vi "High Resolution Wait.vi"(8 "error in (no error)":errorcluster, 11 "wait time (s)":dbl format="%#_6p") -> (0 "error out":errorcluster)   [LabVIEW 2020]
doc: "LabVIEW no longer supports this VI. Use the High Resolution Polling Wait VI instead.\n\nWaits the specified time. Use this VI when you need higher resolution of wait time than you can obtain with the Wait (ms) function. \n\nThe time resolution of this VI may vary with different operating systems and CPU types.\n\nUnlike the Wait (ms) function, this VI does not yield. If <b>wait time</b> is less than 1 to 2 ms, this VI polls in a tight loop. If <b>wait time</b> is greater than 1 to 2 ms, this VI polls in a tight loop for the last 1 to 2 ms."
panel:
  # "This VI is deprecated. Use the following VI instead:\n\nvi.lib\\Utility\\High Resolution Polling Wait.vi"
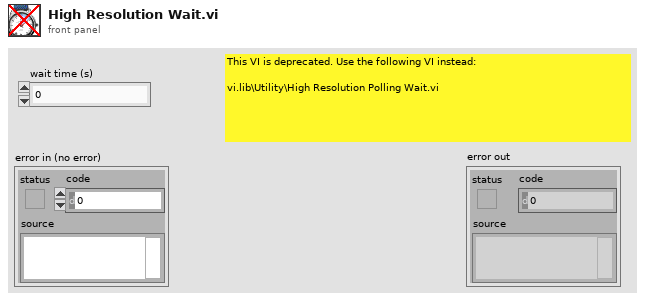
[diagram p1: front panel]
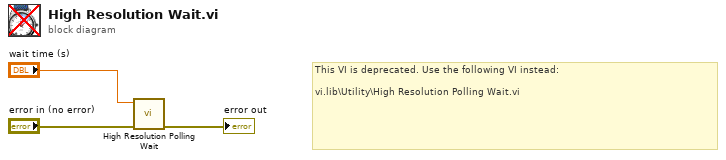
[diagram p0: block diagram]
diagram:
  # "This VI is deprecated. Use the following VI instead:\n\nvi.lib\\Utility\\High Resolution Polling Wait.vi"
  n1 = call <vilib>:"High Resolution Polling Wait.vi"("error in (no error)"="error in (no error)", "seconds to wait"="wait time (s)") -> ("error out"=→"error out":errorcluster)  [unwired: 9 in]
